vi "Write RP transceiver.vi"(8 "error in (no error)":errorcluster, 10 "RP Transceiver.lvclass":refnum<class "RP Transceiver.lvclass">, 11 "Spectrum Recorder too in":refnum<class "Spectrum Recorder too.lvclass">) -> (0 "error out":errorcluster, 3 "Spectrum Recorder too out":refnum<class "Spectrum Recorder too.lvclass">)   [LabVIEW 2018, in "Spectrum Recorder too.lvclass"]
uses:
  Spectrum Recorder too.lvclass
  C:/github/LabActor/Instrument Actor/Instrument Actor.lvclass
  NHMFL_Core/Libraries/Red Pitaya/RP Core/RP Transceiver/RP Transceiver.lvclass
  Instrument Actor/Instrument Actor.lvclass/Instrument Actor.ctl
  NHMFL_Core/Libraries/Red Pitaya/RP Core/Red Pitaya Transceiver Driver/Red Pitaya Transceiver Driver.lvclass
  C:/github/NHMFL_Core/Libraries/Instruments/Instrument Driver/Instrument Driver.lvclass
  NHMFL_Core/Libraries/Red Pitaya/RP Core/Red Pitaya Transceiver Driver/Red Pitaya Transceiver Driver.lvclass/Red Pitaya Transceiver Driver.ctl
  Instrument Actor/Read Instrument driver.vi
  NHMFL_Core/Libraries/Red Pitaya/RP Core/Red Pitaya Transceiver Driver/Write RP Transceiver.vi
  Instrument Actor/Write Instrument driver.vi
  NHMFL_Core/Libraries/Instruments/Instrument Driver/Instrument Driver.lvclass
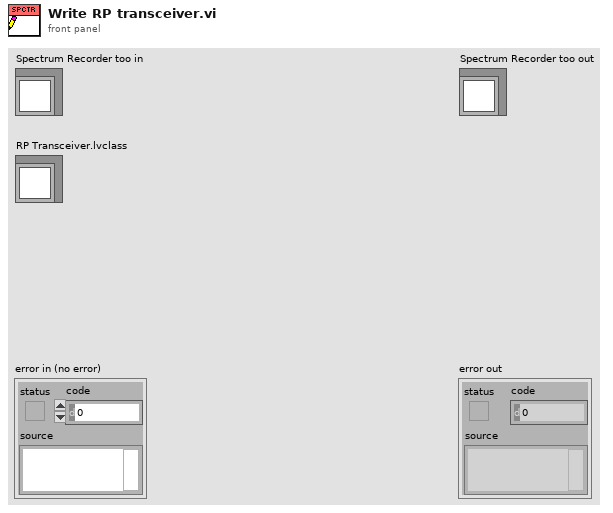
[diagram p1: front panel]
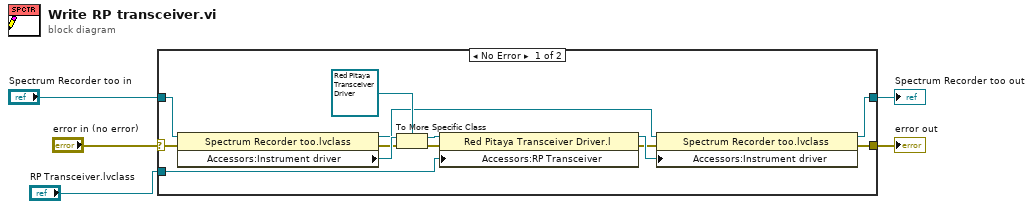
[diagram p0: block diagram]
diagram:
  n1 = case shown="No Error" "error in (no error)" {
    selector: "error in (no error)" -> [w14 w19]
    tunnel: [w6 w19] -> w4
    tunnel: [w7 w20] -> w2
    tunnel: "Spectrum Recorder too in" -> [w18 w20]
    tunnel: "RP Transceiver.lvclass" -> [w10 _]
    frame No Error {
      n2 = property class="Spectrum Recorder too.lvclass"(reference=w18, error in=w14) -> (reference out=w11:refnum<class "Spectrum Recorder too.lvclass">, error out=w13:errorcluster, "Accessors:Instrument driver"=w17:refnum<class "Instrument Driver.lvclass">)
      n3 = To More Specific Class(target class=refnum<class "Red Pitaya Transceiver Driver.lvclass"> refnum ("Red Pitaya Transceiver Driver.lvclass"), reference=w17, error in=w13) -> (specific class reference=w15:refnum<class "Red Pitaya Transceiver Driver.lvclass">, error out=w12:errorcluster)
      n4 = property class="Red Pitaya Transceiver Driver.l"(reference=w15, error in=w12, "Accessors:RP Transceiver"=w10) -> (reference out=w9:refnum<class "Red Pitaya Transceiver Driver.lvclass">, error out=w8:errorcluster)
      n5 = property class="Spectrum Recorder too.lvclass"(reference=w11, error in=w8, "Accessors:Instrument driver"=w9) -> (reference out=w7:refnum<class "Spectrum Recorder too.lvclass">, error out=w6:errorcluster)
    }
    frame Error {
    }
  }
  "error out" <- w4
  "Spectrum Recorder too out" <- w2
